vi "Write Goto (No Objects).vi"(8 "error in (no error)":errorcluster, 9 "Enable warning? (T)":bool=TRUE, 10 "Target":dbl[unit], 11 "Cluster In":T4={"Field"=0.0, "Rate"=0.0, "Status"={"Sweeping"=FALSE, "Clamped"=FALSE, "Hold"=FALSE, "At Rest"=FALSE, "Quench"=FALSE, "Persistent Mode"=FALSE, "Switch Heater"=FALSE}, "ILM Shut Down?"=FALSE, "IO Info"={"Address"={"Com Port"=1, "ISOBUS Address"=2, "GPIB Address"=24, "Communication"=enum."ISOBUS"}, "Version"=enum."IPS"}, "IO Info (Level Meter)"={"Address"={"Com Port"=1, "ISOBUS Address"=5, "GPIB Address"=24, "Communication"=enum."ISOBUS"}, "ILM Name"="", "Display Channel"=[]}, "Training?"=FALSE, "Training Field and Speed Cluster"={"Training Field"=[0.0, 4.108, 5.78, 8.001], "Training Speed"=[0.0057, 0.0022833333333333334, 0.0011333333333333334, 0.0011333333333333334]}}) -> (0 "error out":errorcluster, 3 "Cluster Out":T4={"Field"=0.0, "Rate"=0.0, "Status"={"Sweeping"=FALSE, "Clamped"=FALSE, "Hold"=FALSE, "At Rest"=FALSE, "Quench"=FALSE, "Persistent Mode"=FALSE, "Switch Heater"=FALSE}, "ILM Shut Down?"=FALSE, "IO Info"={"Address"={"Com Port"=1, "ISOBUS Address"=2, "GPIB Address"=24, "Communication"=enum."ISOBUS"}, "Version"=enum."IPS"}, "IO Info (Level Meter)"={"Address"={"Com Port"=1, "ISOBUS Address"=5, "GPIB Address"=24, "Communication"=enum."ISOBUS"}, "ILM Name"="", "Display Channel"=[]}, "Training?"=FALSE, "Training Field and Speed Cluster"={"Training Field"=[0.0, 4.108, 5.78, 8.001], "Training Speed"=[0.0057, 0.0022833333333333334, 0.0011333333333333334, 0.0011333333333333334]}})   [LabVIEW 2012]
doc: "Tells magnet to now go to the target field (if Goto Zero is set to true, goes to 0 instead)."
uses:
  Magnet status.ctl
  Oxford/PSSUBS.LLB/PSIO.ctl
  Oxford/BUSGEN.LLB/OxfordAddress.ctl
  Power Supply.lvclass
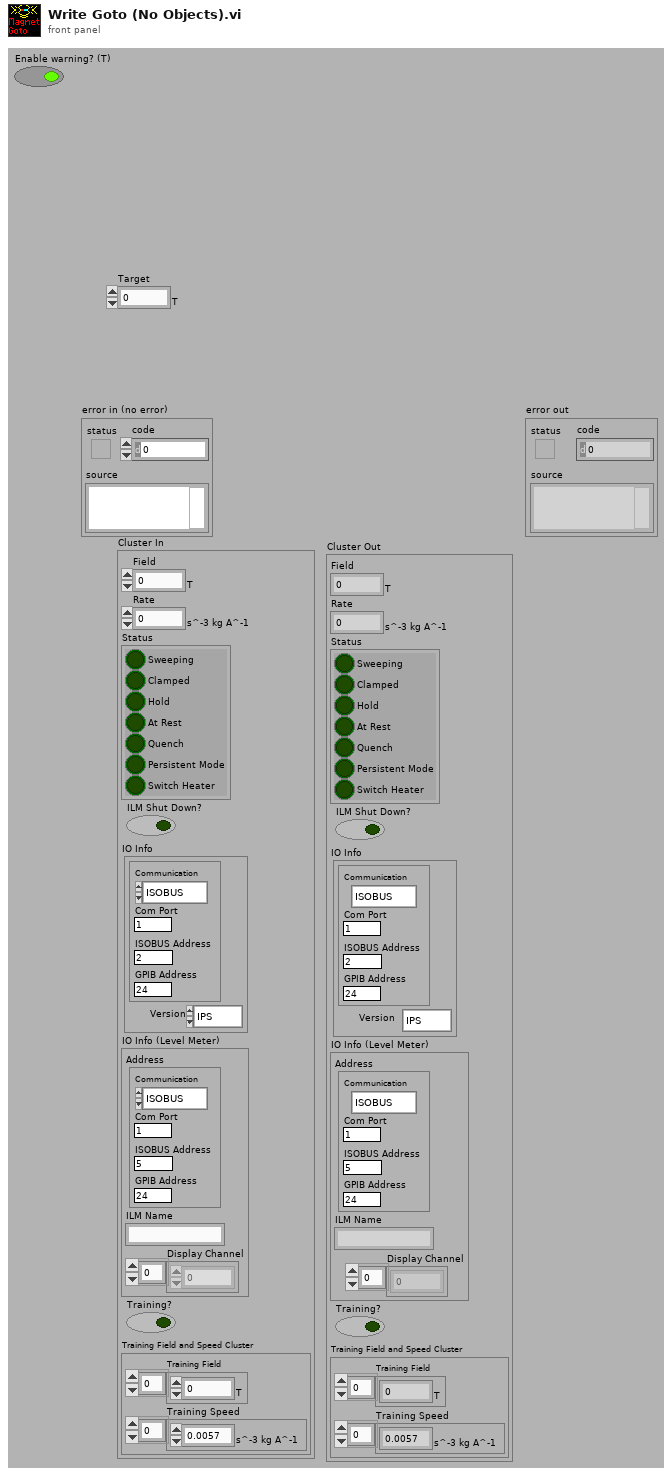
[diagram p1: front panel]
types:
  T1 = typedef "Power Supply.lvclass/Magnet status.ctl" = cluster{"Sweeping":bool, "Clamped":bool, "Hold":bool, "At Rest":bool, "Quench":bool, "Persistent Mode":bool, "Switch Heater":bool}
  T2 = typedef "PSIO.ctl" = cluster{"Address":T3, "Version":enum16{"PS", "IPS"}}
  T3 = typedef "OxfordAddress.ctl" = cluster{"Com Port":i32, "ISOBUS Address":i32, "GPIB Address":i16, "Communication":enum16{"RS232", "ISOBUS", "GPIB", "Gateway"}}
  T4 = cluster{"Field":dbl[unit], "Rate":dbl[unit], "Status":T1, "ILM Shut Down?":bool, "IO Info":T2, "IO Info (Level Meter)":cluster{"Address":T3, "ILM Name":string, "Display Channel":i32[]}, "Training?":bool, "Training Field and Speed Cluster":cluster{"Training Field":dbl[unit][], "Training Speed":dbl[unit][]}}
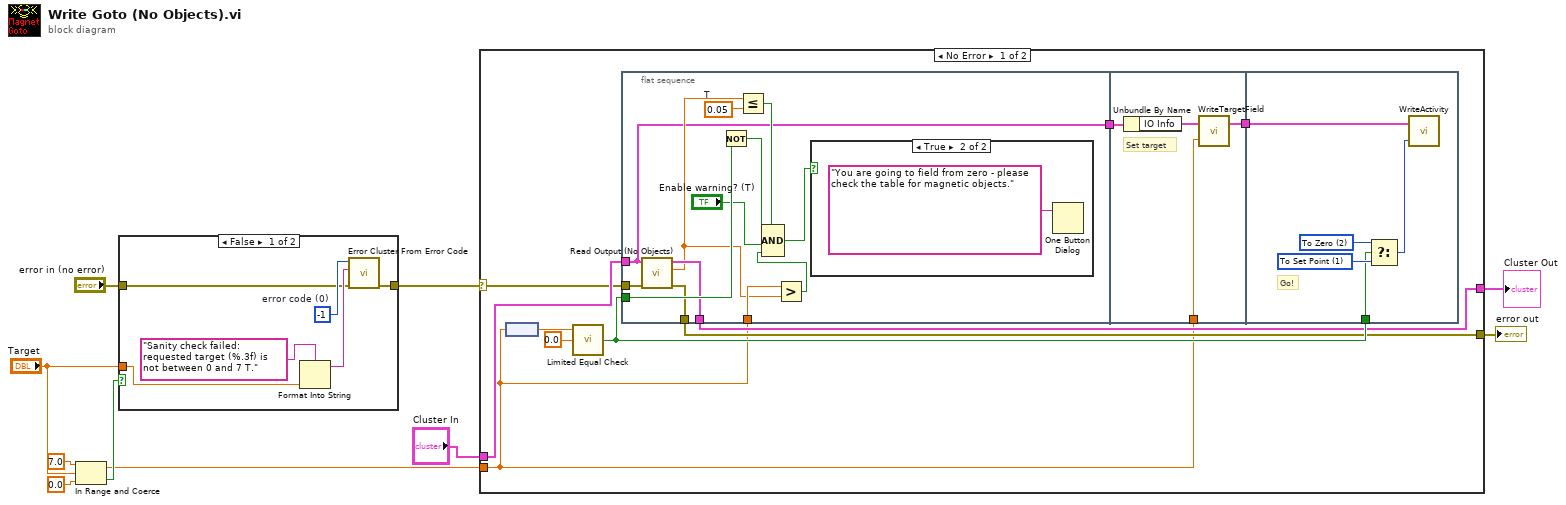
[diagram p0: block diagram]
diagram:
  n1 = In Range and Coerce(upper limit=dbl[unit] 7.0, x="Target", lower limit=dbl[unit] 0.0) -> (coerced(x)=w3:dbl[unit], In Range?=w5:bool)
  n2 = case shown="False" w5 {
    tunnel: [w16 w17] -> w7
    tunnel: "error in (no error)" -> [w11 w17]
    tunnel: "Target" -> [w13 _]
    frame False {
      w15 = -1  # error code (0)
      n3 = Format Into String(format string="Sanity check failed: requested target (%.3f) is not between 0 and 7 T." ("error message (\"\")"), w13) -> (resulting string=w12:string)  [unwired: 2 in, 1 out]
      n4 = call <vilib>:"Error Cluster From Error Code.vi"("error in (no error)"=w11, "error message (\"\")"=w12, "error code (0)"=w15) -> ("error out"=w16:errorcluster)  [unwired: 6 in]
    }
    frame True {
    }
  }
  n5 = case shown="No Error" w7 {
    selector: w7 -> [w20 w51]
    tunnel: "Cluster In" -> [w23 w52]
    tunnel: [w22 w52] -> w1
    tunnel: [w21 w51] -> w10
    tunnel: w3 -> [w18 _]
    frame No Error {
      n6 = node(w18) -> (w19:dbl)
      n7 = call "Limited Equal Check.vi"("number2"=0.0, "number1"=w19) -> ("equal?"=w24:bool)  [unwired: 1 in, 2 out]
      n8 = flat-sequence {
        tunnel: [w28] -> w27
        tunnel: w24 -> [w36]
        tunnel: w23 -> [w28]
        tunnel: [w35] -> w22
        tunnel: w20 -> [w34]
        tunnel: [w33] -> w21
        tunnel: w18 -> [w30]
        tunnel: [w45] -> w26
        tunnel: w27 -> [w44]
        tunnel: w18 -> [w42]
        tunnel: w26 -> [w50]
        tunnel: w24 -> [w46]
        frame #0 {
          w40 = dbl[unit] 0.05  # T
          n9 = call "Read Output (No Objects).vi"("error in (no error)"=w34, "Cluster In"=w28) -> ("error out"=w33:errorcluster, "Field"=w29:dbl[unit], "Cluster Out"=w35:T4)  [unwired: 6 in, 1 out]
          n10 = Not(x=w36) -> (.not. x?=w37:bool)
          n11 = Less Or Equal?(x=w29, y=w40) -> (x <= y?=w39:bool)
          n12 = Greater?(x=w30, y=w29) -> (0:w31:bool)
          n13 = Compound Arithmetic op=AND(w39, w37, "Enable warning? (T)", w31) -> (w38:bool)
          n14 = case shown="True" w38 {
            frame False {
            }
            frame True {
              n15 = One Button Dialog(message="You are going to field from zero - please check the table for magnetic objects.") -> ()  [unwired: 2 out]
            }
          }
        }
        frame #1 {
          # "Set target"
          n16 = Unbundle By Name(w44) -> ("IO Info"=w43:T2)
          n17 = call "WriteTargetField.vi"("Target Field"=w42, "IO Info"=w43) -> ("IO Info"=w45:T2)  [unwired: 1 out]
        }
        frame #2 {
          w47 = u16 2 items=["Hold", "To Set Point", "To Zero", "Clamp"] ("Activity")
          w49 = u16 1 items=["Hold", "To Set Point", "To Zero", "Clamp"] ("Activity")
          # "Go!"
          n18 = Select(t=w47, s=w46, f=w49) -> (s? t:f=w48:u16)
          n19 = call "WriteActivity.vi"("Activity"=w48, "IO Info"=w50) -> ()  [unwired: 2 out]
        }
      }
    }
    frame Error {
    }
  }
  "error out" <- w10
  "Cluster Out" <- w1
